vi "gentec-SOLO_PE.Test.vi"(8 "error in (no error)":errorcluster, 11 "VISA Refnum in":refnum<visa-resource-name>) -> (0 "error out":errorcluster, 1 "Acknoledged?":bool, 2 "Error":string, 3 "VISA Refnum out":refnum<visa-resource-name>, 4 "Timeout":bool)   [LabVIEW 2014, in "gentec-SOLO-PE - Driver.lvlib"]
doc: "This is a simple test VI: It sends a test command to the device, waits a certain time, and reads the data published by the device."
uses:
  gentec-SOLO-PE - Driver.lvlib
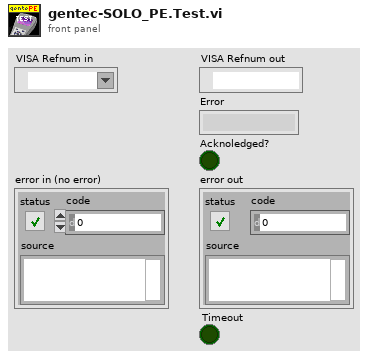
[diagram p1: front panel]
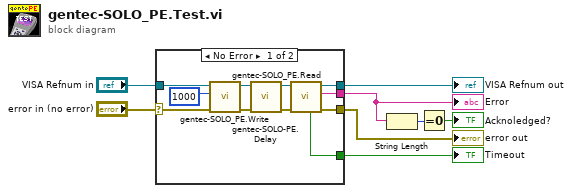
[diagram p0: block diagram]
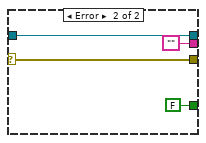
[diagram p2: hidden frame]
diagram:
  n1 = case shown="No Error" "error in (no error)" {
    selector: "error in (no error)" -> [w9 w22]
    tunnel: [w19 w22] -> w8
    tunnel: [w18 w23] -> w7
    tunnel: [w17 FALSE ("Timeout")] -> w6
    tunnel: "VISA Refnum in" -> [w12 w23]
    tunnel: [w10 ""] -> w3
    frame No Error {
      n2 = call "gentec-SOLO_PE.Write.vi"("error in (no error)"=w9, "Command Handle"=u16 1000, "VISA Refnum in"=w12) -> ("error out"=w15:errorcluster, "VISA Refnum out"=w13:refnum<visa-resource-name>)  [unwired: 7 in]
      n3 = call "gentec-SOLO-PE.Delay.vi"("error in (no error)"=w15, "VISA resource In"=w13) -> ("error out"=w16:errorcluster, "VISA resource Out"=w14:refnum<visa-resource-name>)  [unwired: 4 in]
      n4 = call "gentec-SOLO_PE.Read.vi"("error in (no error)"=w16, "VISA Refnum in"=w14) -> ("error out"=w19:errorcluster, "Error"=w10:string, "VISA Refnum out"=w18:refnum<visa-resource-name>, "Timeout"=w17:bool)  [unwired: 5 in, 1 out]
    }
    frame Error {
    }
  }
  "error out" <- w8
  "VISA Refnum out" <- w7
  "Error" <- w3
  "Timeout" <- w6
  n5 = String Length(string=w3) -> (length=w4:i32)
  n6 = Equal To 0?(x=w4) -> (x = 0?=→"Acknoledged?":bool)
